vi "DualDigitalOscilloscope.vi"() -> ()   [LabVIEW 2015]
panel:
  out "error out":errorcluster
  in  "Digitizing Parameters":T1
  in  "stop":bool
  out "Waveform Graph":dynamicdata(graph)
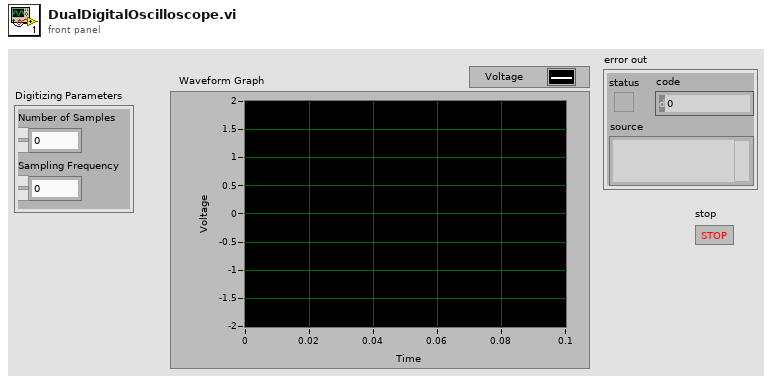
[diagram p1: front panel]
types:
  T1 = cluster{"Number of Samples":dbl, "Sampling Frequency":dbl}
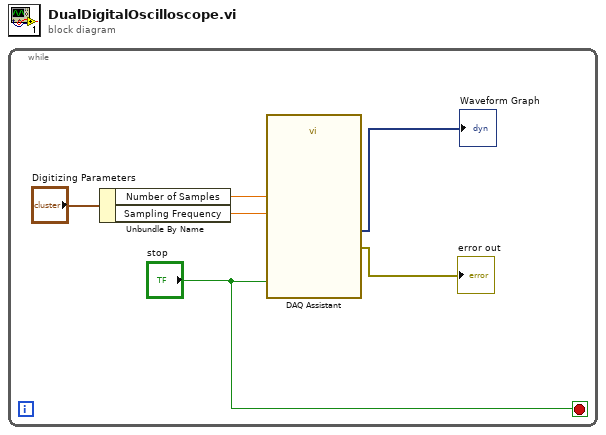
[diagram p0: block diagram]
diagram:
  n1 = while {
    stop <- "stop" stop-if-true
    n2 = Unbundle By Name("Digitizing Parameters") -> ("Number of Samples"=w3:dbl, "Sampling Frequency"=w2:dbl)
    n3 = call "DAQ Assistant"("rate"=w2, "number of samples"=w3, "stop (T)"="stop") -> ("data"=→"Waveform Graph":dynamicdata, "error out"=→"error out":errorcluster)  [unwired: 14 in, 1 out]
  }
